vi "MGI RWA Handle Path.vi"(7 "Conversion":T1, 8 "error in (no error)":errorcluster, 10 "Path data as string":string, 11 "Path":path) -> (0 "error out":errorcluster, 3 "String":string)   [LabVIEW 2020]
uses:
  <userlib>/_MGI/Read Write Anything/MGI RWA Convertion Direction Enum.ctl
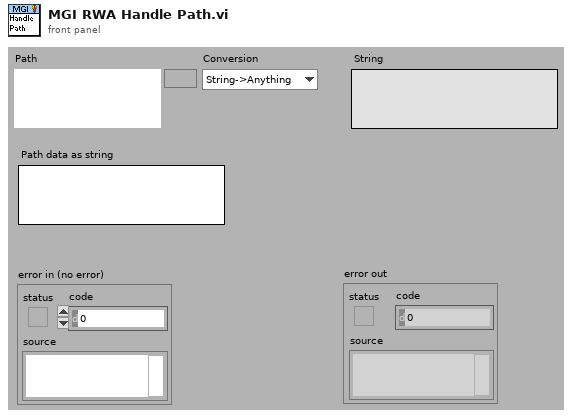
[diagram p1: front panel]
types:
  T1 = typedef "MGI RWA Convertion Direction Enum.ctl" = enum16{"String->Anything", "Anything->String"}
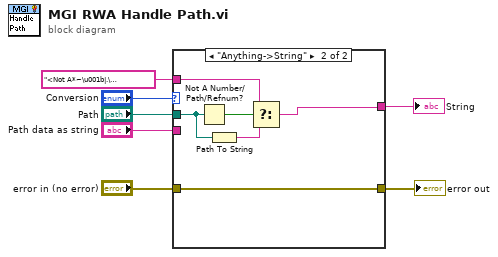
[diagram p0: block diagram]
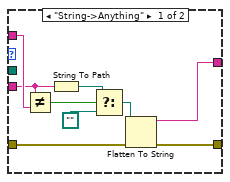
[diagram p2: hidden frame]
diagram:
  n1 = case shown="\"Anything->String\"" "Conversion" {
    tunnel: "error in (no error)" -> [w16 w19]
    tunnel: "Path data as string" -> [w11 _]
    tunnel: "Path" -> [_ w18]
    tunnel: [w15 w19] -> w3
    tunnel: [w14 w20] -> w2
    tunnel: "<Not A*~\u001b|.\u0017Path>" -> [w13 w21]
    frame "String->Anything" {
      n2 = Not Equal?(x=w11, y=w13) -> (x != y?=w12:bool)
      n3 = String To Path(string=w11) -> (path=w10:path)
      n4 = Select(t=w10, s=w12, f=path "") -> (s? t:f=w9:path)
      n5 = Flatten To String(anything=w9, error in (no error)=w16) -> (data string=w14:string, error out=w15:errorcluster)  [unwired: 2 in, 1 out]
    }
    frame "Anything->String" {
      n6 = Not A Number/Path/Refnum?(number/path/refnum=w18) -> (NaN/Path/Refnum?=w22:bool)
      n7 = Path To String(path=w18) -> (string=w17:string)
      n8 = Select(t=w21, s=w22, f=w17) -> (s? t:f=w20:string)
    }
  }
  "String" <- w2
  "error out" <- w3
